vi "Card_detection.vi"(8 "error in (no error)":errorcluster, 10 "Card":bool, 11 "User_Console_States in":refnum<class "User_Console_States.lvclass">) -> (0 "error out":errorcluster, 3 "State out":refnum<class "State Actor.lvclass">)   [LabVIEW 2025, in "User_Console-ATM.lvlib" / "User_Console_States.lvclass"]
uses:
  User_Console_States.lvclass
  C:/Program Files (x86)/National Instruments/LabVIEW 2025/vi.lib/ni/Actors/State Actor/State Actor/State Actor.lvclass
  <vilib>/ni/Actors/State Actor/State Actor/State Actor.lvclass
  User_Console_States.lvclass/User_Console_States.ctl
  C:/Program Files (x86)/National Instruments/LabVIEW 2025/vi.lib/ActorFramework/Actor/Actor.lvclass
  C:/Users/halstead_rideriver/Documents/Labview_Practice/ATM_Machine_Actor Framework/ATM_ACTORFW/User_Console-ATM/User_Console_States/User_Console_States.lvclass
  Card_detection/Card_detection.lvclass
  C:/Users/halstead_rideriver/Documents/Labview_Practice/ATM_Machine_Actor Framework/ATM_ACTORFW/User_Console-ATM/Card_detection/Card_detection.lvclass
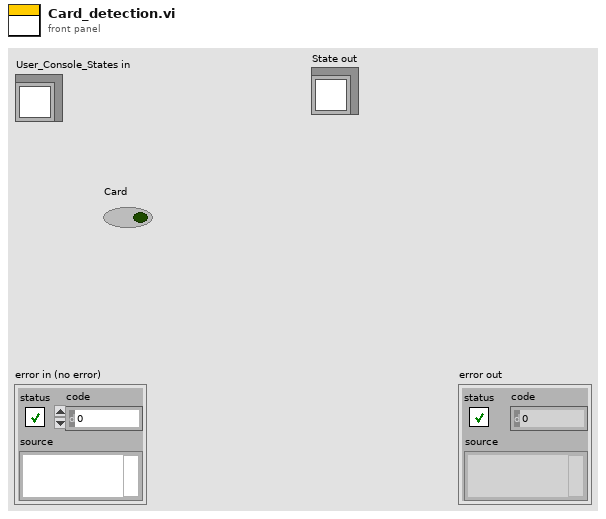
[diagram p1: front panel]
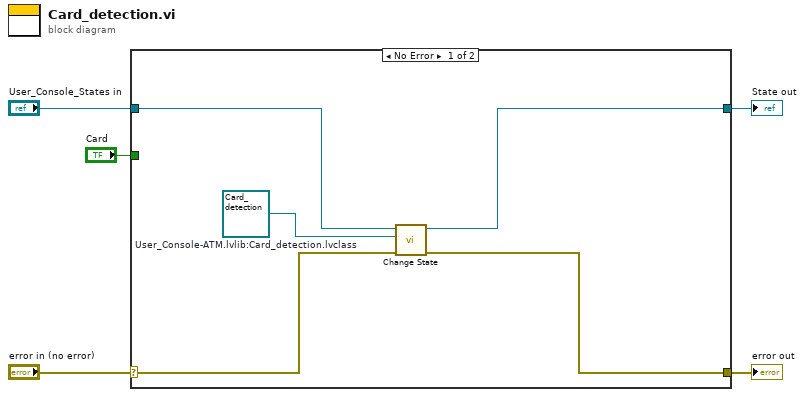
[diagram p0: block diagram]
diagram:
  n1 = case shown="No Error" "error in (no error)" {
    selector: "error in (no error)" -> [w10 w12]
    tunnel: [w9 w12] -> w4
    tunnel: [w8 w11] -> w2
    tunnel: "User_Console_States in" -> [w7 w11]
    tunnel: "Card" -> [_ _]
    frame No Error {
      w6 = refnum<class "Card_detection.lvclass"> refnum  # User_Console-ATM.lvlib:Card_detection.lvclass
      n2 = call <vilib>:"Change State.vi"("error in (no error)"=w10, "New State in"=w6, "State in"=w7) -> ("error out"=w9:errorcluster, "State out"=w8:refnum<class "State Actor.lvclass">)  [unwired: 7 in]
    }
    frame Error {
    }
  }
  "error out" <- w4
  "State out" <- w2
